vi "save_data.vi"() -> ()   [LabVIEW 2023]
uses:
  <vilib>/Utility/NIReport.llb/Report Type.ctl
  global_variables.vi
  <vilib>/Utility/NIReport.llb/Append Text Table to Report (wrap).vi
  <vilib>/Utility/NIReport.llb/NI_report.lvclass
  <vilib>/Utility/NIReport.llb/NI_ReportGenerationCore.lvlib
  <vilib>/Utility/NIReport.llb/Excel/NI_Excel.lvclass
panel:
  in  "load_from_file":bool
  in  "request_to_server":bool
  in  "acquisition_from_arduino":bool
  in  "help_button":bool
  in  "close_button":bool
  in  "SAVE_RING":u16(ring) items=["Click and Choose", "All Data Report .TXT", "All Data Report .XLSX", "Temperature Report .TXT", "Temperature Report .XLSX", "Perceived temp. Report .TXT", "Perceived temp. Report .XLSX", "Humidity Report .TXT", "Humidity Report .XLSX"]
  # "SAVE DATA"
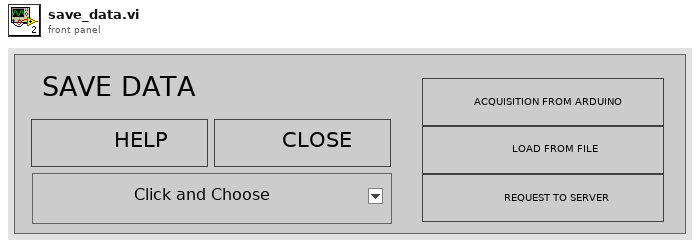
[diagram p1: front panel]
types:
  T1 = enum16{"open", "replace", "create", "open or create", "replace or create", "replace or create with confirmation"}
  T2 = typedef "NI_ReportGenerationCore.lvlib/Report Type.ctl" = enum16{"HTML", "Word", "Excel"}
  T3 = enum32{"Invalid", "Standard", "Closed", "Hidden", "Minimized", "Maximized"}
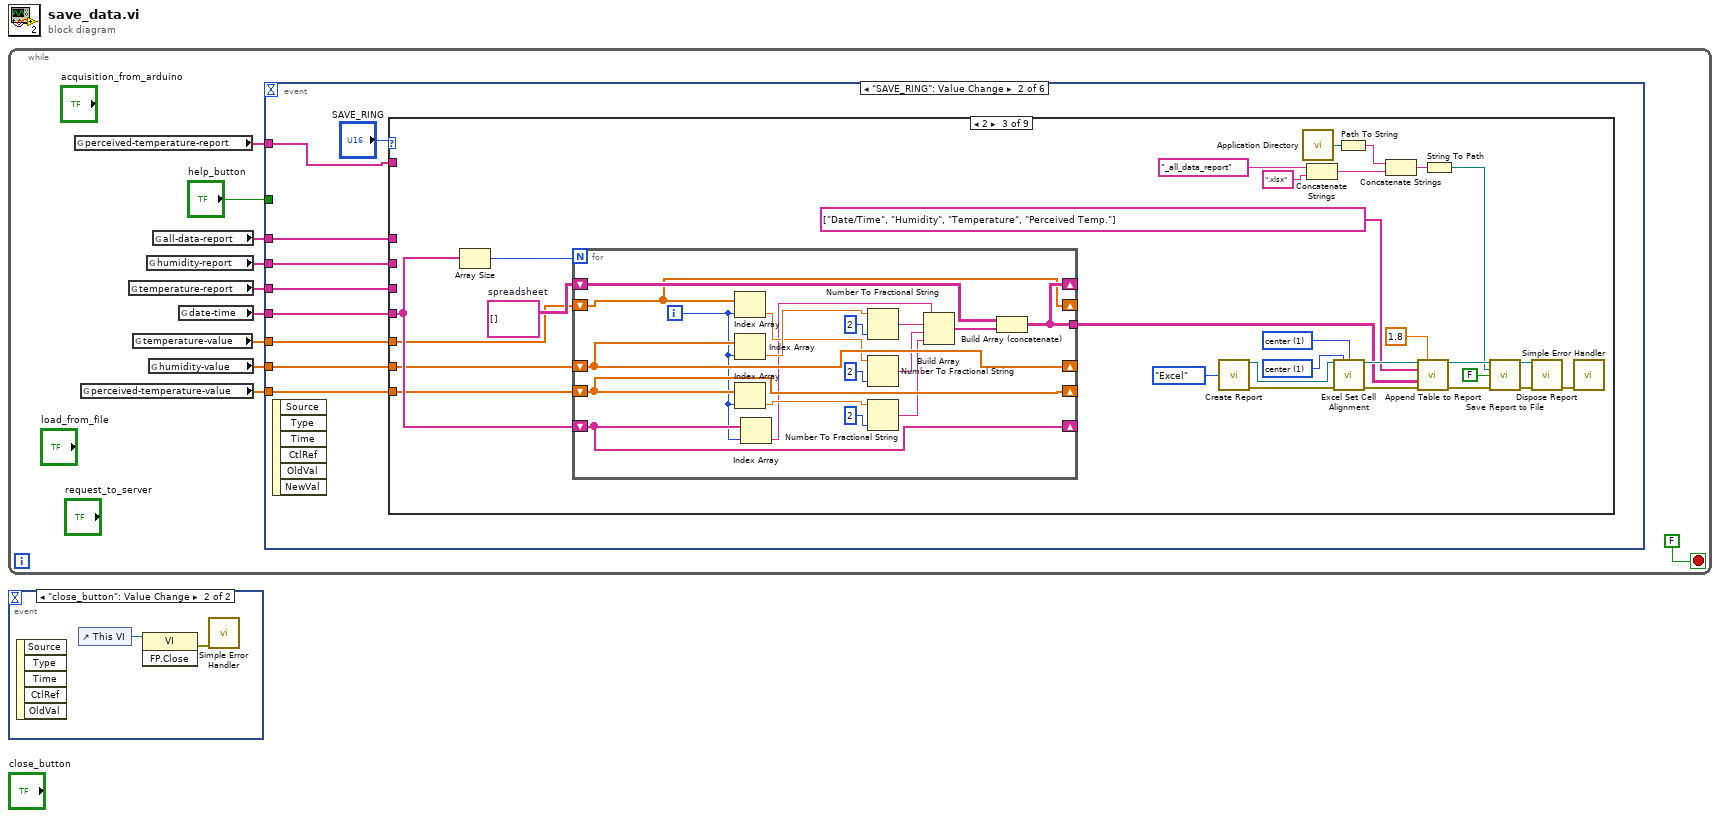
[diagram p0: block diagram]
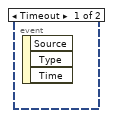
[diagram p2: hidden frame]
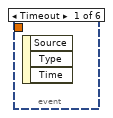
[diagram p3: hidden frame]
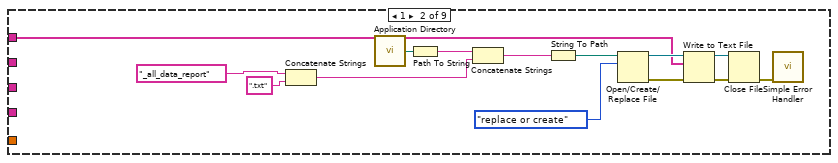
[diagram p5: hidden frame]
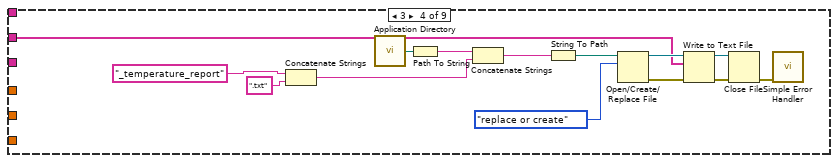
[diagram p6: hidden frame]
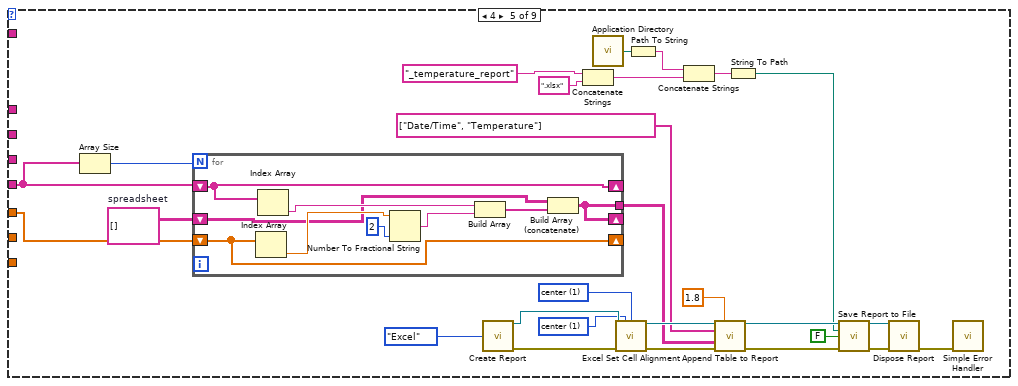
[diagram p7: hidden frame]
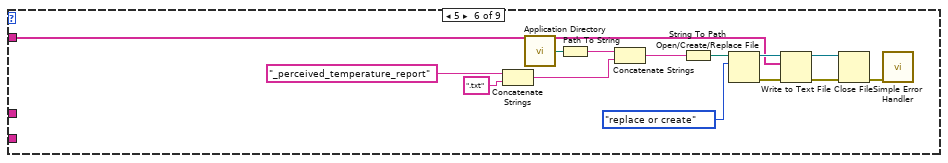
[diagram p8: hidden frame]
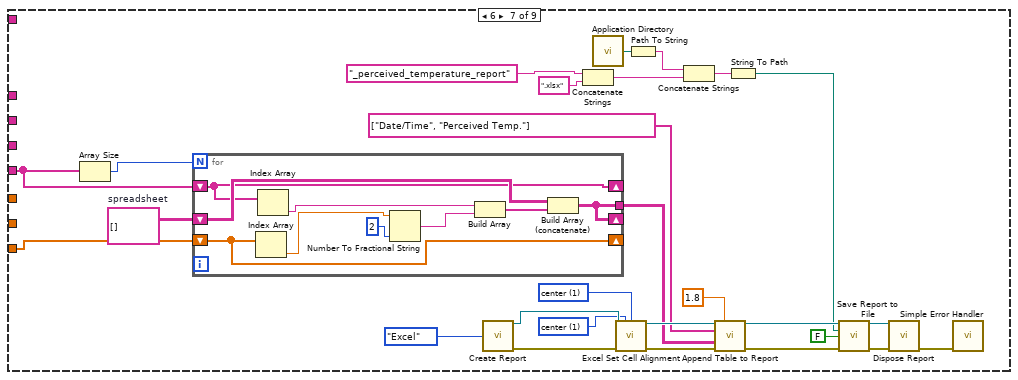
[diagram p9: hidden frame]
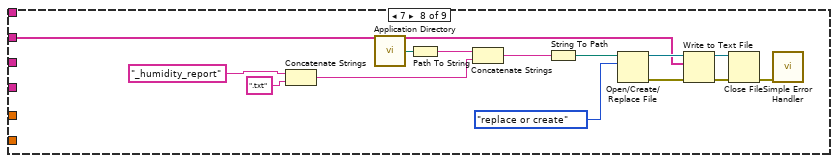
[diagram p10: hidden frame]
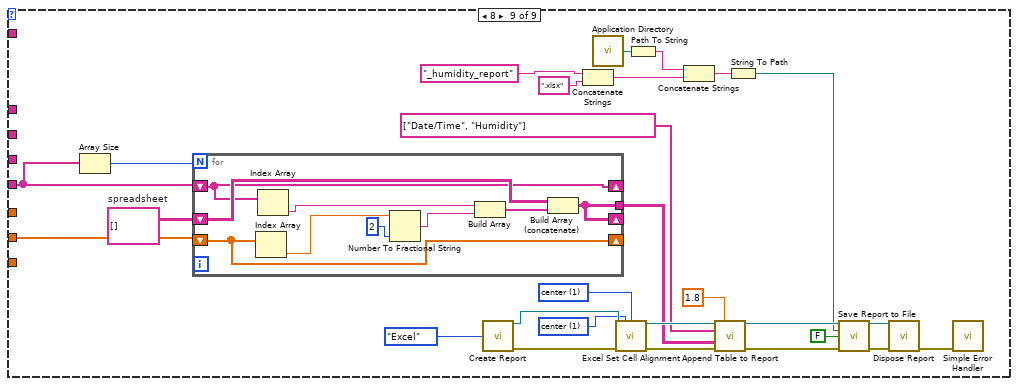
[diagram p11: hidden frame]
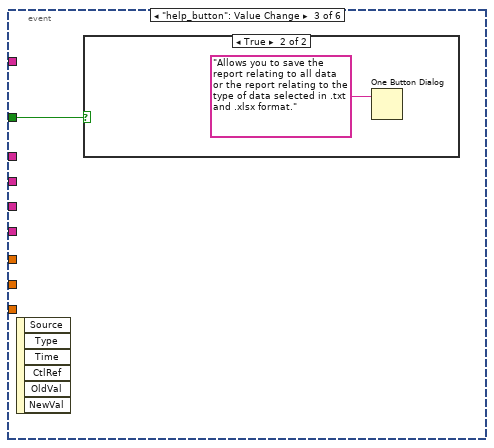
[diagram p12: hidden frame]
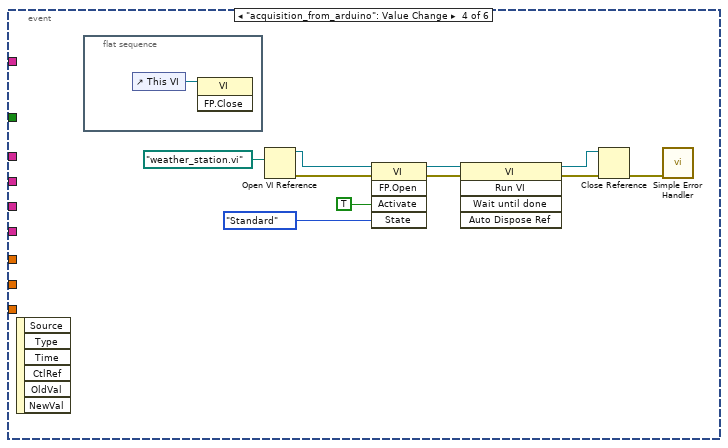
[diagram p14: hidden frame]
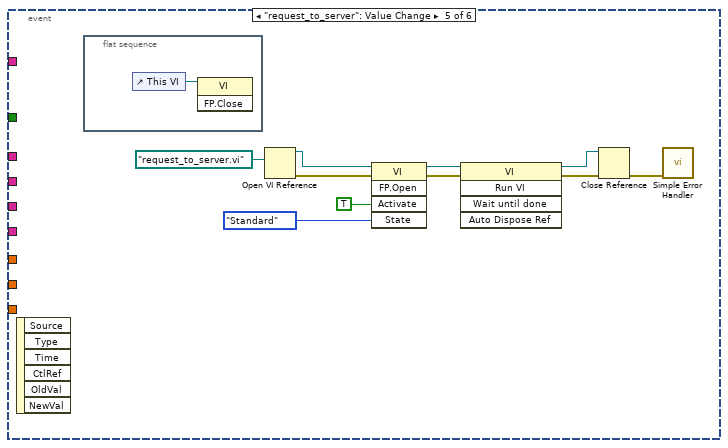
[diagram p15: hidden frame]
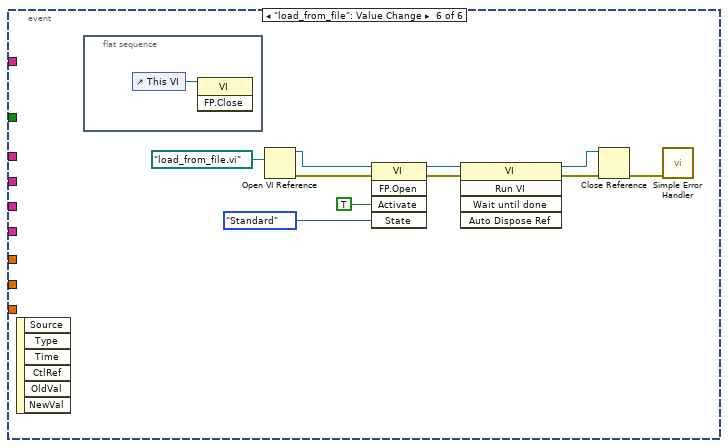
[diagram p16: hidden frame]
diagram:
  n1 = while {
    stop <- FALSE stop-if-true
    n2 = global read "global_variables.vi" "perceived-temperature-report"() -> (w3:string[])
    n3 = global read "global_variables.vi" "perceived-temperature-value"() -> (w6:dbl[])
    n4 = global read "global_variables.vi" "temperature-report"() -> (w5:string[])
    n5 = global read "global_variables.vi" "temperature-value"() -> (w8:dbl[])
    n6 = global read "global_variables.vi" "humidity-report"() -> (w4:string[])
    n7 = global read "global_variables.vi" "humidity-value"() -> (w7:dbl[])
    n8 = global read "global_variables.vi" "all-data-report"() -> (w10:string[])
    n9 = global read "global_variables.vi" "date-time"() -> (w9:string[])
    n10 = event shown="[1] \"SAVE_RING\": Value Change" {
      selector: _ -> [_ _ _ _ _ _]
      dyn-events: _ -> [_ _ _ _ _ _]
      timeout: _ -> [_ _ _ _ _ _]
      tunnel: w10 -> [_ w19 _ _ _ _]
      tunnel: w9 -> [_ w18 _ _ _ _]
      tunnel: w8 -> [_ w17 _ _ _ _]
      tunnel: w7 -> [_ w16 _ _ _ _]
      tunnel: w6 -> [_ w15 _ _ _ _]
      tunnel: w5 -> [_ w14 _ _ _ _]
      tunnel: w4 -> [_ w13 _ _ _ _]
      tunnel: w3 -> [_ w12 _ _ _ _]
      tunnel: "help_button" -> [_ _ w231 _ _ _]
      event Timeout {
        n11 = event-data() -> ()  [unwired: 1 in, 3 out]
      }
      event "SAVE_RING": Value Change {
        n12 = event-data() -> ()  [unwired: 1 in, 6 out]
        n13 = case shown="2" "SAVE_RING" {
          tunnel: w19 -> [_ w20 _ _ _ _ _ _ _]
          tunnel: w18 -> [_ _ w37 _ w96 _ w146 _ w196]
          tunnel: w17 -> [_ _ w34 _ w95 _ _ _ _]
          tunnel: w16 -> [_ _ w35 _ _ _ _ _ w195]
          tunnel: w15 -> [_ _ w36 _ _ _ w145 _ _]
          tunnel: w14 -> [_ _ _ w81 _ _ _ _ _]
          tunnel: w13 -> [_ _ _ _ _ _ _ w181 _]
          tunnel: w12 -> [_ _ _ _ _ w131 _ _ _]
          frame 0, Default {
          }
          frame 1 {
            n14 = Concatenate Strings("_all_data_report" ("string"), ".txt") -> (w27:string)
            n15 = call <vilib>:"Application Directory.vi"() -> ("Application Directory"=w23:path)
            n16 = Path To String(path=w23) -> (string=w24:string)
            n17 = Concatenate Strings(w24, w27) -> (w22:string)
            n18 = String To Path(string=w22) -> (path=w26:path)
            n19 = Open/Create/Replace File(file path (use dialog)=w26, operation (0:open)=T1."replace or create") -> (refnum out=w31:refnum<file>, error out=w30:errorcluster)  [unwired: 4 in, 1 out]
            n20 = Write to Text File(file (use dialog)=w31, text=w20, error in=w30) -> (refnum out=w33:refnum<file>, error out=w32:errorcluster)  [unwired: 1 in, 1 out]
            n21 = Close File(refnum=w33, error in=w32) -> (error out=w21:errorcluster)  [unwired: 1 out]
            n22 = call <vilib>:"Simple Error Handler.vi"("error in (no error)"=w21) -> ()  [unwired: 4 in, 5 out]
          }
          frame 2 {
            w43 = string[][] []  # spreadsheet
            w58 = 1 items=["left", "center", "right"] ("horizontal alignment (left)")
            w59 = 1 items=["top", "center", "bottom"] ("vertical alignment (top)")
            n23 = Array Size(array=w37) -> (size(s)=w44:i32)
            n24 = for {
              N: w44 -> [_]
              shift-right: [w75] -> _
              shift-left: w37 -> [w75]
              shift-right: [w80] -> _
              shift-left: w35 -> [w80]
              shift-right: [w66] -> _
              shift-left: w34 -> [w66]
              shift-right: [w76] -> _
              shift-left: w36 -> [w76]
              shift-right: [w72] -> _
              shift-left: w43 -> [w73]
              tunnel: [w72] -> w42
              i -> [w70]
              n25 = Index Array(array=w66, index=w70) -> (element=w78:dbl)
              n26 = Index Array(array=w80, index=w70) -> (element=w79:dbl)
              n27 = Index Array(array=w76, index=w70) -> (element=w77:dbl)
              n28 = Index Array(array=w75, index=w70) -> (element=w74:string)
              n29 = Number To Fractional String(number=w79, precision (6)=i16 2) -> (F-format string=w69:string)  [unwired: 2 in]
              n30 = Number To Fractional String(number=w78, precision (6)=i16 2) -> (F-format string=w68:string)  [unwired: 2 in]
              n31 = Number To Fractional String(number=w77, precision (6)=i16 2) -> (F-format string=w67:string)  [unwired: 2 in]
              n32 = Build Array(w74, w69, w68, w67) -> (w71:string[])
              n33 = Build Array (concatenate)(w73, w71) -> (w72:string[][])
            }
            n34 = call <vilib>:"Create Report.vi"("report type"=Report_Type."Excel") -> ("report out"=w61:refnum<class "NI_report.lvclass">, "error out"=w60:errorcluster)  [unwired: 13 in]
            n35 = call <vilib>:"Application Directory.vi"() -> ("Application Directory"=w48:path)
            n36 = Concatenate Strings("_all_data_report" ("string"), ".xlsx") -> (w51:string)
            n37 = call <vilib>:"Excel Set Cell Alignment.vi"("report in"=w61, "vertical alignment (top)"=w59, "horizontal alignment (left)"=w58, "error in (no error)"=w60) -> ("report out"=w57:refnum<class "NI_report.lvclass">, "error out"=w56:errorcluster)  [unwired: 10 in]
            n38 = Path To String(path=w48) -> (string=w49:string)
            n39 = Concatenate Strings(w49, w51) -> (w47:string)
            n40 = call-poly <vilib>:"Append Table to Report.vi"("report in"=w57, "column width (1)"=1.8, "column headers"=string[] ["Date/Time", "Humidity", "Temperature", "Perceived Temp."], "text data"=w42, "error in (no error)"=w56) -> ("report out"=w55:refnum<class "NI_report.lvclass">, "error out"=w54:errorcluster)  [unwired: 7 in, 2 out]
            n41 = String To Path(string=w47) -> (path=w46:path)
            n42 = call-dynamic "Save Report to File.vi"("report in"=w55, "report file path"=w46, "prompt to replace? (F)"=FALSE, "error in (no error)"=w54) -> ("report out"=w53:refnum<class "NI_report.lvclass">, "error out"=w52:errorcluster)  [unwired: 10 in]
            n43 = call-dynamic "Dispose Report.vi"("report in"=w53, "error in (no error)"=w52) -> ("error out"=w39:errorcluster)  [unwired: 13 in]
            n44 = call <vilib>:"Simple Error Handler.vi"("error in (no error)"=w39) -> ()  [unwired: 4 in, 5 out]
          }
          frame 3 {
            n45 = Concatenate Strings("_temperature_report" ("string"), ".txt") -> (w88:string)
            n46 = call <vilib>:"Application Directory.vi"() -> ("Application Directory"=w84:path)
            n47 = Path To String(path=w84) -> (string=w85:string)
            n48 = Concatenate Strings(w85, w88) -> (w83:string)
            n49 = String To Path(string=w83) -> (path=w87:path)
            n50 = Open/Create/Replace File(file path (use dialog)=w87, operation (0:open)=T1."replace or create") -> (refnum out=w92:refnum<file>, error out=w91:errorcluster)  [unwired: 4 in, 1 out]
            n51 = Write to Text File(file (use dialog)=w92, text=w81, error in=w91) -> (refnum out=w94:refnum<file>, error out=w93:errorcluster)  [unwired: 1 in, 1 out]
            n52 = Close File(refnum=w94, error in=w93) -> (error out=w82:errorcluster)  [unwired: 1 out]
            n53 = call <vilib>:"Simple Error Handler.vi"("error in (no error)"=w82) -> ()  [unwired: 4 in, 5 out]
          }
          frame 4 {
            w107 = string[][] []  # spreadsheet
            w118 = 1 items=["left", "center", "right"] ("horizontal alignment (left)")
            w119 = 1 items=["top", "center", "bottom"] ("vertical alignment (top)")
            n54 = Array Size(array=w96) -> (size(s)=w106:i32)
            n55 = for {
              N: w106 -> [_]
              shift-right: [w123] -> _
              shift-left: w107 -> [w127]
              shift-right: [w125] -> _
              shift-left: w96 -> [w125]
              shift-right: [w124] -> _
              shift-left: w95 -> [w124]
              tunnel: [w123] -> w105
              n56 = Index Array(array=w124) -> (element=w128:dbl)  [unwired: 1 in]
              n57 = Index Array(array=w125) -> (element=w130:string)  [unwired: 1 in]
              n58 = Number To Fractional String(number=w128, precision (6)=i16 2) -> (F-format string=w129:string)  [unwired: 2 in]
              n59 = Build Array(w130, w129) -> (w126:string[])
              n60 = Build Array (concatenate)(w127, w126) -> (w123:string[][])
            }
            n61 = call <vilib>:"Create Report.vi"("report type"=Report_Type."Excel") -> ("report out"=w120:refnum<class "NI_report.lvclass">, "error out"=w103:errorcluster)  [unwired: 13 in]
            n62 = Concatenate Strings("_temperature_report" ("string"), ".xlsx") -> (w114:string)
            n63 = call <vilib>:"Application Directory.vi"() -> ("Application Directory"=w111:path)
            n64 = call <vilib>:"Excel Set Cell Alignment.vi"("report in"=w120, "vertical alignment (top)"=w119, "horizontal alignment (left)"=w118, "error in (no error)"=w103) -> ("report out"=w117:refnum<class "NI_report.lvclass">, "error out"=w102:errorcluster)  [unwired: 10 in]
            n65 = Path To String(path=w111) -> (string=w112:string)
            n66 = Concatenate Strings(w112, w114) -> (w110:string)
            n67 = call-poly <vilib>:"Append Table to Report.vi"("report in"=w117, "column width (1)"=1.8, "column headers"=string[] ["Date/Time", "Temperature"], "text data"=w105, "error in (no error)"=w102) -> ("report out"=w116:refnum<class "NI_report.lvclass">, "error out"=w101:errorcluster)  [unwired: 7 in, 2 out]
            n68 = String To Path(string=w110) -> (path=w109:path)
            n69 = call-dynamic "Save Report to File.vi"("report in"=w116, "report file path"=w109, "prompt to replace? (F)"=FALSE, "error in (no error)"=w101) -> ("report out"=w115:refnum<class "NI_report.lvclass">, "error out"=w100:errorcluster)  [unwired: 10 in]
            n70 = call-dynamic "Dispose Report.vi"("report in"=w115, "error in (no error)"=w100) -> ("error out"=w98:errorcluster)  [unwired: 13 in]
            n71 = call <vilib>:"Simple Error Handler.vi"("error in (no error)"=w98) -> ()  [unwired: 4 in, 5 out]
          }
          frame 5 {
            n72 = Concatenate Strings("_perceived_temperature_report" ("string"), ".txt") -> (w138:string)
            n73 = call <vilib>:"Application Directory.vi"() -> ("Application Directory"=w134:path)
            n74 = Path To String(path=w134) -> (string=w135:string)
            n75 = Concatenate Strings(w135, w138) -> (w133:string)
            n76 = String To Path(string=w133) -> (path=w137:path)
            n77 = Open/Create/Replace File(file path (use dialog)=w137, operation (0:open)=T1."replace or create") -> (refnum out=w142:refnum<file>, error out=w141:errorcluster)  [unwired: 4 in, 1 out]
            n78 = Write to Text File(file (use dialog)=w142, text=w131, error in=w141) -> (refnum out=w144:refnum<file>, error out=w143:errorcluster)  [unwired: 1 in, 1 out]
            n79 = Close File(refnum=w144, error in=w143) -> (error out=w132:errorcluster)  [unwired: 1 out]
            n80 = call <vilib>:"Simple Error Handler.vi"("error in (no error)"=w132) -> ()  [unwired: 4 in, 5 out]
          }
          frame 6 {
            w156 = string[][] []  # spreadsheet
            w168 = 1 items=["left", "center", "right"] ("horizontal alignment (left)")
            w169 = 1 items=["top", "center", "bottom"] ("vertical alignment (top)")
            n81 = Array Size(array=w146) -> (size(s)=w157:i32)
            n82 = for {
              N: w157 -> [_]
              shift-right: [w175] -> _
              shift-left: w156 -> [w180]
              shift-right: [w174] -> _
              shift-left: w146 -> [w174]
              shift-right: [w173] -> _
              shift-left: w145 -> [w173]
              tunnel: [w175] -> w155
              n83 = Index Array(array=w173) -> (element=w179:dbl)  [unwired: 1 in]
              n84 = Index Array(array=w174) -> (element=w176:string)  [unwired: 1 in]
              n85 = Number To Fractional String(number=w179, precision (6)=i16 2) -> (F-format string=w177:string)  [unwired: 2 in]
              n86 = Build Array(w176, w177) -> (w178:string[])
              n87 = Build Array (concatenate)(w180, w178) -> (w175:string[][])
            }
            n88 = call <vilib>:"Create Report.vi"("report type"=Report_Type."Excel") -> ("report out"=w170:refnum<class "NI_report.lvclass">, "error out"=w150:errorcluster)  [unwired: 13 in]
            n89 = Concatenate Strings("_perceived_temperature_report" ("string"), ".xlsx") -> (w164:string)
            n90 = call <vilib>:"Application Directory.vi"() -> ("Application Directory"=w161:path)
            n91 = call <vilib>:"Excel Set Cell Alignment.vi"("report in"=w170, "vertical alignment (top)"=w169, "horizontal alignment (left)"=w168, "error in (no error)"=w150) -> ("report out"=w167:refnum<class "NI_report.lvclass">, "error out"=w151:errorcluster)  [unwired: 10 in]
            n92 = Path To String(path=w161) -> (string=w162:string)
            n93 = Concatenate Strings(w162, w164) -> (w160:string)
            n94 = call-poly <vilib>:"Append Table to Report.vi"("report in"=w167, "column width (1)"=1.8, "column headers"=string[] ["Date/Time", "Perceived Temp."], "text data"=w155, "error in (no error)"=w151) -> ("report out"=w166:refnum<class "NI_report.lvclass">, "error out"=w153:errorcluster)  [unwired: 7 in, 2 out]
            n95 = String To Path(string=w160) -> (path=w159:path)
            n96 = call-dynamic "Save Report to File.vi"("report in"=w166, "report file path"=w159, "prompt to replace? (F)"=FALSE, "error in (no error)"=w153) -> ("report out"=w165:refnum<class "NI_report.lvclass">, "error out"=w152:errorcluster)  [unwired: 10 in]
            n97 = call-dynamic "Dispose Report.vi"("report in"=w165, "error in (no error)"=w152) -> ("error out"=w148:errorcluster)  [unwired: 13 in]
            n98 = call <vilib>:"Simple Error Handler.vi"("error in (no error)"=w148) -> ()  [unwired: 4 in, 5 out]
          }
          frame 7 {
            n99 = Concatenate Strings("_humidity_report" ("string"), ".txt") -> (w188:string)
            n100 = call <vilib>:"Application Directory.vi"() -> ("Application Directory"=w184:path)
            n101 = Path To String(path=w184) -> (string=w185:string)
            n102 = Concatenate Strings(w185, w188) -> (w183:string)
            n103 = String To Path(string=w183) -> (path=w187:path)
            n104 = Open/Create/Replace File(file path (use dialog)=w187, operation (0:open)=T1."replace or create") -> (refnum out=w192:refnum<file>, error out=w191:errorcluster)  [unwired: 4 in, 1 out]
            n105 = Write to Text File(file (use dialog)=w192, text=w181, error in=w191) -> (refnum out=w194:refnum<file>, error out=w193:errorcluster)  [unwired: 1 in, 1 out]
            n106 = Close File(refnum=w194, error in=w193) -> (error out=w182:errorcluster)  [unwired: 1 out]
            n107 = call <vilib>:"Simple Error Handler.vi"("error in (no error)"=w182) -> ()  [unwired: 4 in, 5 out]
          }
          frame 8 {
            w206 = string[][] []  # spreadsheet
            w218 = 1 items=["left", "center", "right"] ("horizontal alignment (left)")
            w219 = 1 items=["top", "center", "bottom"] ("vertical alignment (top)")
            n108 = Array Size(array=w196) -> (size(s)=w207:i32)
            n109 = for {
              N: w207 -> [_]
              shift-right: [w225] -> _
              shift-left: w206 -> [w230]
              shift-right: [w224] -> _
              shift-left: w196 -> [w224]
              shift-right: [w223] -> _
              shift-left: w195 -> [w223]
              tunnel: [w225] -> w205
              n110 = Index Array(array=w223) -> (element=w229:dbl)  [unwired: 1 in]
              n111 = Index Array(array=w224) -> (element=w226:string)  [unwired: 1 in]
              n112 = Number To Fractional String(number=w229, precision (6)=i16 2) -> (F-format string=w227:string)  [unwired: 2 in]
              n113 = Build Array(w226, w227) -> (w228:string[])
              n114 = Build Array (concatenate)(w230, w228) -> (w225:string[][])
            }
            n115 = call <vilib>:"Create Report.vi"("report type"=Report_Type."Excel") -> ("report out"=w220:refnum<class "NI_report.lvclass">, "error out"=w203:errorcluster)  [unwired: 13 in]
            n116 = Concatenate Strings("_humidity_report" ("string"), ".xlsx") -> (w214:string)
            n117 = call <vilib>:"Application Directory.vi"() -> ("Application Directory"=w211:path)
            n118 = call <vilib>:"Excel Set Cell Alignment.vi"("report in"=w220, "vertical alignment (top)"=w219, "horizontal alignment (left)"=w218, "error in (no error)"=w203) -> ("report out"=w217:refnum<class "NI_report.lvclass">, "error out"=w202:errorcluster)  [unwired: 10 in]
            n119 = Path To String(path=w211) -> (string=w212:string)
            n120 = Concatenate Strings(w212, w214) -> (w210:string)
            n121 = call-poly <vilib>:"Append Table to Report.vi"("report in"=w217, "column width (1)"=1.8, "column headers"=string[] ["Date/Time", "Humidity"], "text data"=w205, "error in (no error)"=w202) -> ("report out"=w216:refnum<class "NI_report.lvclass">, "error out"=w201:errorcluster)  [unwired: 7 in, 2 out]
            n122 = String To Path(string=w210) -> (path=w209:path)
            n123 = call-dynamic "Save Report to File.vi"("report in"=w216, "report file path"=w209, "prompt to replace? (F)"=FALSE, "error in (no error)"=w201) -> ("report out"=w215:refnum<class "NI_report.lvclass">, "error out"=w200:errorcluster)  [unwired: 10 in]
            n124 = call-dynamic "Dispose Report.vi"("report in"=w215, "error in (no error)"=w200) -> ("error out"=w198:errorcluster)  [unwired: 13 in]
            n125 = call <vilib>:"Simple Error Handler.vi"("error in (no error)"=w198) -> ()  [unwired: 4 in, 5 out]
          }
        }
      }
      event "help_button": Value Change {
        n126 = event-data() -> ()  [unwired: 1 in, 6 out]
        n127 = case shown="True" w231 {
          frame False {
          }
          frame True {
            n128 = One Button Dialog(message="Allows you to save the report relating to all data or the report relating to the type of data selected in .txt and .xlsx format.") -> ()  [unwired: 1 in, 1 out]
          }
        }
      }
      event "acquisition_from_arduino": Value Change {
        n129 = event-data() -> ()  [unwired: 1 in, 6 out]
        n130 = flat-sequence {
          frame #0 {
            n131 = control-ref of="This VI"() -> (w243:refnum<vi>)
            n132 = invoke class="VI" method="FP.Close"(reference=w243) -> ()  [unwired: 2 in, 3 out]
          }
        }
        n133 = Open VI Reference(vi path=path "weather_station.vi") -> (vi reference=w236:refnum<vi>, error out=w237:errorcluster)  [unwired: 5 in]
        n134 = invoke class="VI" method="FP.Open"(reference=w236, error in=w237, "Activate"=TRUE ("Activate?"), "State"=T3."Standard") -> (reference out=w238:refnum<vi>, error out=w239:errorcluster)  [unwired: 1 in, 3 out]
        n135 = invoke class="VI" method="Run VI"(reference=w238, error in=w239) -> (reference out=w241:refnum<vi>, error out=w240:errorcluster)  [unwired: 3 in, 3 out]
        n136 = Close Reference(reference=w241, error in (no error)=w240) -> (error out=w242:errorcluster)
        n137 = call <vilib>:"Simple Error Handler.vi"("error in (no error)"=w242) -> ()  [unwired: 4 in, 5 out]
      }
      event "request_to_server": Value Change {
        n138 = event-data() -> ()  [unwired: 1 in, 6 out]
        n139 = flat-sequence {
          frame #0 {
            n140 = control-ref of="This VI"() -> (w254:refnum<vi>)
            n141 = invoke class="VI" method="FP.Close"(reference=w254) -> ()  [unwired: 2 in, 3 out]
          }
        }
        n142 = Open VI Reference(vi path=path "request_to_server.vi") -> (vi reference=w247:refnum<vi>, error out=w248:errorcluster)  [unwired: 5 in]
        n143 = invoke class="VI" method="FP.Open"(reference=w247, error in=w248, "Activate"=TRUE ("Activate?"), "State"=T3."Standard") -> (reference out=w249:refnum<vi>, error out=w250:errorcluster)  [unwired: 1 in, 3 out]
        n144 = invoke class="VI" method="Run VI"(reference=w249, error in=w250) -> (reference out=w252:refnum<vi>, error out=w251:errorcluster)  [unwired: 3 in, 3 out]
        n145 = Close Reference(reference=w252, error in (no error)=w251) -> (error out=w253:errorcluster)
        n146 = call <vilib>:"Simple Error Handler.vi"("error in (no error)"=w253) -> ()  [unwired: 4 in, 5 out]
      }
      event "load_from_file": Value Change {
        n147 = event-data() -> ()  [unwired: 1 in, 6 out]
        n148 = flat-sequence {
          frame #0 {
            n149 = control-ref of="This VI"() -> (w265:refnum<vi>)
            n150 = invoke class="VI" method="FP.Close"(reference=w265) -> ()  [unwired: 2 in, 3 out]
          }
        }
        n151 = Open VI Reference(vi path=path "load_from_file.vi") -> (vi reference=w258:refnum<vi>, error out=w259:errorcluster)  [unwired: 5 in]
        n152 = invoke class="VI" method="FP.Open"(reference=w258, error in=w259, "Activate"=TRUE ("Activate?"), "State"=T3."Standard") -> (reference out=w260:refnum<vi>, error out=w261:errorcluster)  [unwired: 1 in, 3 out]
        n153 = invoke class="VI" method="Run VI"(reference=w260, error in=w261) -> (reference out=w263:refnum<vi>, error out=w262:errorcluster)  [unwired: 3 in, 3 out]
        n154 = Close Reference(reference=w263, error in (no error)=w262) -> (error out=w264:errorcluster)
        n155 = call <vilib>:"Simple Error Handler.vi"("error in (no error)"=w264) -> ()  [unwired: 4 in, 5 out]
      }
    }
  }
  n156 = event shown="[1] \"close_button\": Value Change" {
    selector: _ -> [_ _]
    dyn-events: _ -> [_ _]
    timeout: _ -> [_ _]
    event Timeout {
      n157 = event-data() -> ()  [unwired: 1 in, 3 out]
    }
    event "close_button": Value Change {
      n158 = event-data() -> ()  [unwired: 1 in, 5 out]
      n159 = control-ref of="This VI"() -> (w267:refnum<vi>)
      n160 = invoke class="VI" method="FP.Close"(reference=w267) -> (error out=w266:errorcluster)  [unwired: 2 in, 2 out]
      n161 = call <vilib>:"Simple Error Handler.vi"("error in (no error)"=w266) -> ()  [unwired: 4 in, 5 out]
    }
  }
